vi "flow pressure sensor.vi"() -> ()   [LabVIEW 2014]
uses:
  <vilib>/MakerHub/LINX/Public/Peripherals/Analog/Analog Read N Chans.vi
  <vilib>/MakerHub/LINX/Private/Local IO/LinxAnalogRead.vi
  <vilib>/MakerHub/LINX/Public/Utilities/Check Channel.vi
  <vilib>/MakerHub/LINX/Private/Utilties/Generate Error.vi
  <vilib>/addons/control/pid/pid.llb/PID Control Input Filter (DBL).vi
  <vilib>/MakerHub/LINX/LMH-LINX.lvlib
  <vilib>/addons/control/pid/NI_PID_pid.lvlib
panel:
  in  "Serial Port":refnum<visa-resource-name>="N/A"
  out "System Error":bool=TRUE
  out "Flowrate Sensor 2":dbl format="%#_13g"
  out "Flowrate Sensor 1":dbl format="%#_13g"
  out "Pressure 2":dbl format="%#_13g"
  out "Pressure 1":dbl format="%#_13g"
  out "Error Message":string
  out "Stop":bool=TRUE
  out "Pressure Chart":T1(graph)
  out "Flowrate Chart":T1(graph)
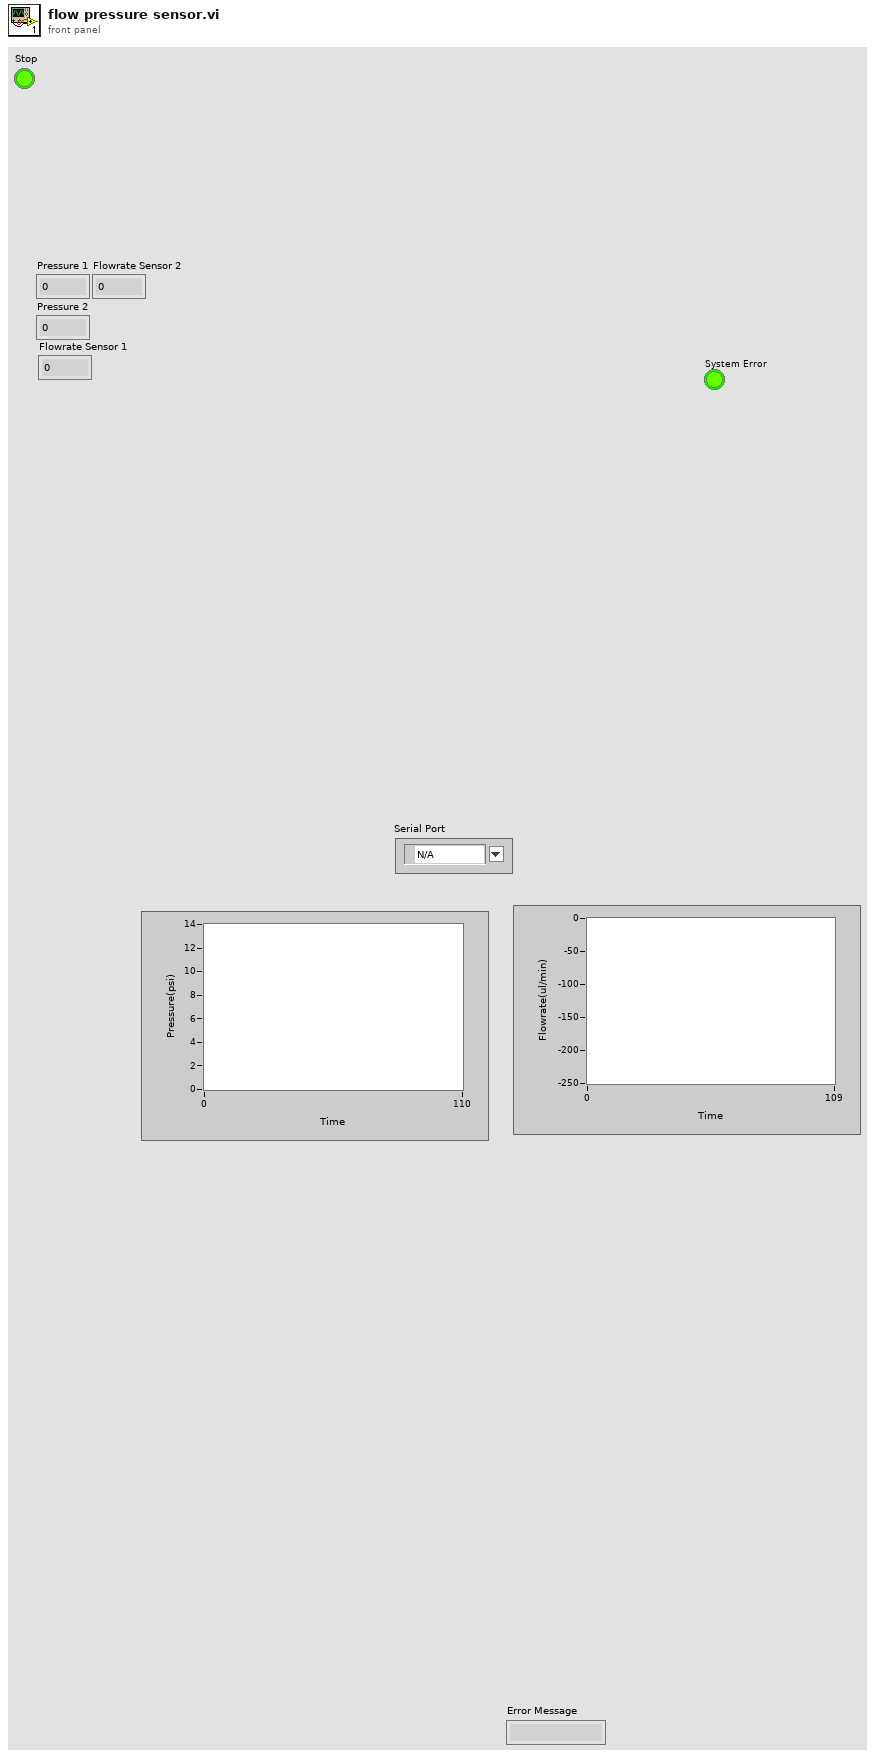
[diagram p1: front panel]
types:
  T1 = cluster{"[0]":dbl, "[1]":dbl, "[2]":dbl, "[3]":dbl, "[4]":dbl, "[5]":dbl, "[6]":dbl, "[7]":dbl, "[8]":dbl}
  T2 = typedef "LMH-LINX.lvlib/LINX Ref.ctl" = cluster{"IO":T3, "Interface":T4, "LINX Device Config":T5}
  T3 = typedef "LMH-LINX.lvlib/Platform.ctl" = enum16{"Remote", "Local"}
  T4 = typedef "LMH-LINX.lvlib/Interface.ctl" = enum16{"Serial", "TCP"}
  T5 = typedef "LMH-LINX.lvlib/Device.lvlib/LINX Device Config.ctl" = cluster{"Interface":T4, "COM Port":refnum<visa-resource-name>, "TCP Configuration":T6, "Device Family":u8, "Device ID":u8, "Device Name":string, "TCP Ref":refnum<k5>, "Channels":T7}
  T6 = typedef "LMH-LINX.lvlib/Device.lvlib/TCP Config.ctl" = cluster{"IP Address":string, "Port":u16}
  T7 = typedef "LMH-LINX.lvlib/Channels.ctl" = cluster{"DI":u8[], "DO":u8[], "AI":u8[], "AO":u8[], "PWM":u8[], "QE":u8[], "UART":u8[], "I2C 2":u8[], "SPI":u8[], "CAN":u8[], "Servo":u8[], "AI Ref (V)":dbl, "AI Resolution (Bits)":u8, "AO Ref (V)":dbl, "AO Resolution (Bits)":u8}
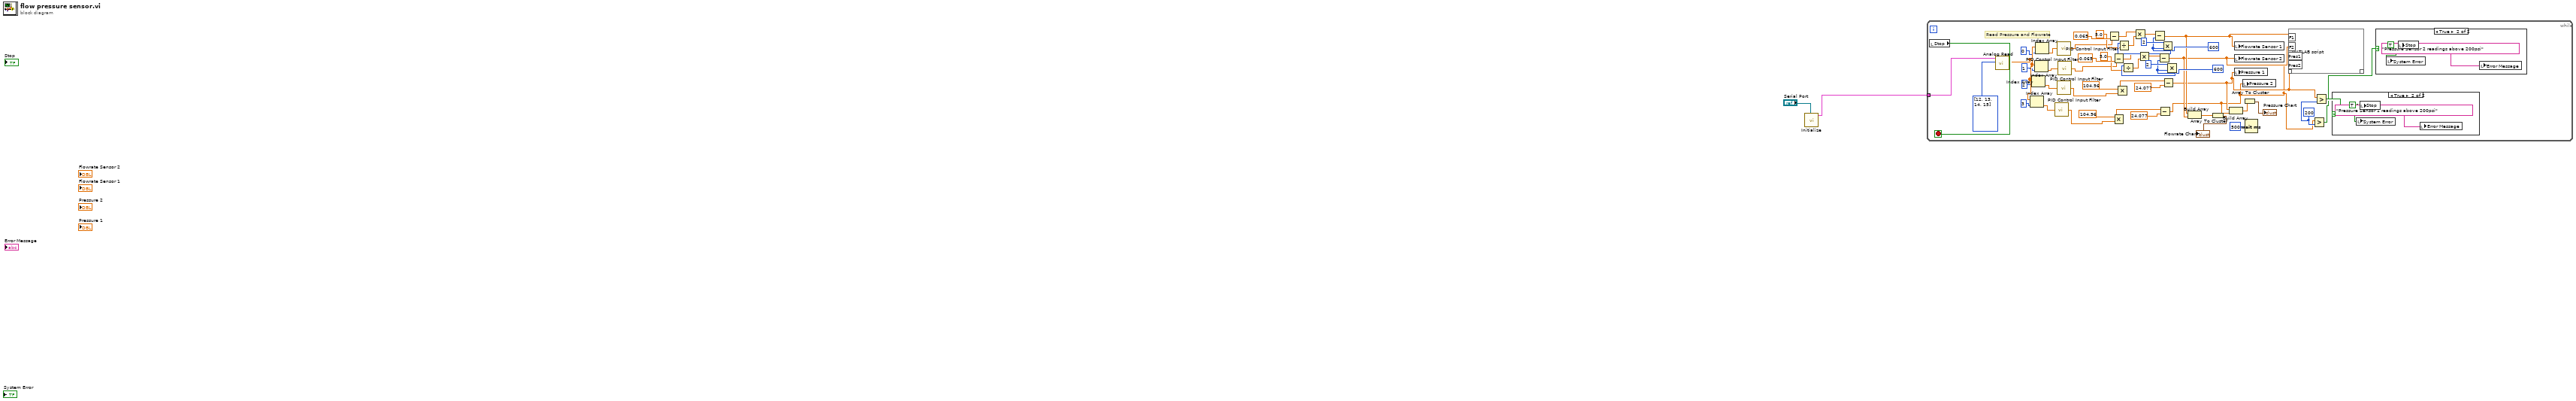
[diagram p0: block diagram]
diagram:
  n1 = call <vilib>:"Initialize.vi"("Serial Port"="Serial Port") -> ("LINX Resource"=w2:T2)  [unwired: 8 in, 2 out]
  n2 = while {
    tunnel: w2 -> [w51]
    stop <- w52 stop-if-true
    w7 = 200
    w18 = 600
    w27 = 600
    # "Read Pressure and Flowrate"
    n3 = local read "Stop"() -> (w52:bool)
    n4 = call-poly <vilib>:"Analog Read.vi"("AI Channel(s)"=i32[] [12, 13, 14, 15], "LINX Resource"=w51) -> ("Voltages"=w49:dbl[])  [unwired: 6 in, 3 out]
    n5 = Index Array(array=w49, index=3) -> (element=w41:dbl)
    n6 = Index Array(array=w49, index=2) -> (element=w42:dbl)
    n7 = Index Array(array=w49, index=1) -> (element=w43:dbl)
    n8 = Index Array(array=w49, index=0) -> (element=w44:dbl)
    n9 = call-poly <vilib>:"PID Control Input Filter.vi"("input"=w41) -> ("output"=w34:dbl)  [unwired: 4 in]
    n10 = call-poly <vilib>:"PID Control Input Filter.vi"("input"=w42) -> ("output"=w33:dbl)  [unwired: 4 in]
    n11 = call-poly <vilib>:"PID Control Input Filter.vi"("input"=w44) -> ("output"=w23:dbl)  [unwired: 4 in]
    n12 = call-poly <vilib>:"PID Control Input Filter.vi"("input"=w43) -> ("output"=w14:dbl)  [unwired: 4 in]
    n13 = Subtract(x=w23, y=0.065) -> (x-y=w24:dbl)
    n14 = Subtract(x=w14, y=0.065) -> (x-y=w15:dbl)
    n15 = Multiply(x=104.96 ("y"), y=w34) -> (x*y=w35:dbl)
    n16 = Multiply(x=104.96 ("y"), y=w33) -> (x*y=w38:dbl)
    n17 = Subtract(x=w35, y=24.077) -> (x-y=w5:dbl)
    n18 = Multiply(x=2, y=w27) -> (x*y=w29:i32)
    n19 = Divide(x=w29, y=5.0) -> (x/y=w25:dbl)
    n20 = Multiply(x=w24, y=w25) -> (x*y=w26:dbl)
    n21 = Subtract(x=w26, y=w27) -> (x-y=w9:dbl)
    n22 = Subtract(x=w38, y=24.077) -> (x-y=w6:dbl)
    n23 = Multiply(x=2, y=w18) -> (x*y=w20:i32)
    n24 = Divide(x=w20, y=5.0) -> (x/y=w16:dbl)
    n25 = Multiply(x=w15, y=w16) -> (x*y=w17:dbl)
    n26 = Subtract(x=w17, y=w18) -> (x-y=w8:dbl)
    n27 = Build Array(w9, w8) -> (w12:dbl[])
    n28 = Array To Cluster(array=w12) -> (cluster=→"Flowrate Chart":T1)
    n29 = Build Array(w6, w5) -> (w13:dbl[])
    n30 = local write "Flowrate Sensor 1"(w9) -> ()
    n31 = local write "Flowrate Sensor 2"(w8) -> ()
    n32 = local write "Pressure 1"(w6) -> ()
    n33 = local write "Pressure 2"(w5) -> ()
    n34 = Array To Cluster(array=w13) -> (cluster=→"Pressure Chart":T1)
    n35 = Wait (ms)(milliseconds to wait=u32 500) -> ()  [unwired: 1 out]
    n36 = script code="MATLAB script"("F1"=w9, "F2"=w8, "Pres1"=w6, "Pres2"=w5) -> ()  [unwired: 1 in, 1 out]
    n37 = Greater?(x=w5, y=w7) -> (0:w3:bool)
    n38 = Greater?(x=w6, y=w7) -> (0:w4:bool)
    n39 = case shown="True" w4 {
      frame False {
      }
      frame True {
        w56 = TRUE ("Stop")
        n40 = local write "System Error"(w56) -> ()
        n41 = local write "Stop"(w56) -> ()
        n42 = local write "Error Message"("Pressure Sensor 1 readings above 200psi") -> ()
      }
    }
    n43 = case shown="True" w3 {
      frame False {
      }
      frame True {
        w54 = TRUE ("Stop")
        n44 = local write "System Error"(w54) -> ()
        n45 = local write "Stop"(w54) -> ()
        n46 = local write "Error Message"("Pressure Sensor 2 readings above 200psi") -> ()
      }
    }
  }
